vi "niScope Query Trigger Edge.vi"(0 "instrument handle":refnum<k15>, 11 "error in":errorcluster {"code" format="%.0x"}) -> (2 "trigger coupling":i32(slide)=1, 3 "trigger slope":i32(slide), 4 "instrument handle out":refnum<k15>, 6 "trigger source":string(combo)="VAL_IMMEDIATE", 8 "trigger level":dbl format="%.2f", 13 "trigger delay":dbl format="%.4f", 14 "trigger holdoff":dbl format="%.4f", 15 "error out":errorcluster {"code" format="%.0x"})   [LabVIEW 2011]
doc: "This VI configures the common properties of the trigger subsystem. \n\nWhen you call niScope Read Waveform or niScope Initiate Acquisition, the oscilloscope waits for a trigger. You specify the type of trigger for which the oscilloscope waits with the Trigger Type parameter. You specify the source the oscilloscope monitors for the trigger with the Trigger Source parameter. After the oscilloscope receives the trigger, the oscilloscope waits the length of time you specify with the Trigger Delay parameter and then marks this spot as the Reference. The value you specify with the Reference Position parameter of niScope Configure Horizontal determines where the Reference is positioned in a record relative to the start of that record.\n\nIf the oscilloscope is configured to acquire multiple records, it waits the length of time specified with Trigger Holdoff after each record before the trigger system is set to trigger for the next record.\n\nNotes:\n(1) After you call this function, you must call the trigger configuration VI that corresponds to the Trigger Type you select to completely specify the trigger. These configuration functions are niScope Configure Digital Trigger, niScope Configure Edge Trigger, niScope Configure Hysteresis Trigger, niScope Configure TV Trigger, and niScope Configure Window Trigger."
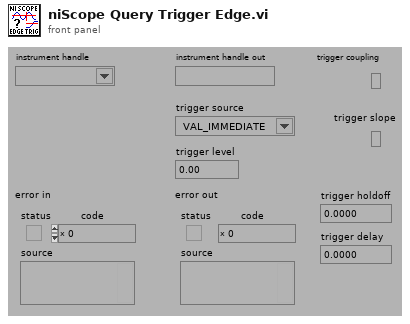
[diagram p1: front panel]
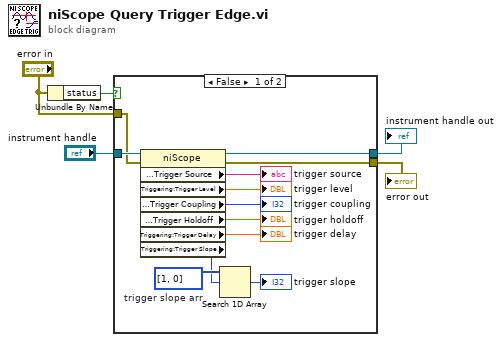
[diagram p0: block diagram]
diagram:
  n1 = Unbundle By Name("error in") -> ("status"=w4:bool)
  n2 = case shown="False" w4 {
    tunnel: "error in" -> [w16 w19]
    tunnel: [w7 w19] -> w3
    tunnel: "instrument handle" -> [w17 w18]
    tunnel: [w6 w18] -> w1
    frame False {
      w15 = i32[] [1, 0]  # trigger slope arr
      n3 = property class="niScope"(reference=w17, error in=w16) -> (reference out=w6:refnum<k15>, error out=w7:errorcluster, "Triggering:Trigger Source"=→"trigger source":string, "Triggering:Trigger Level"=→"trigger level":dbl, "Triggering:Trigger Coupling"=→"trigger coupling":i32, "Triggering:Trigger Holdoff"=→"trigger holdoff":dbl, "Triggering:Trigger Delay"=→"trigger delay":dbl, "Triggering:Trigger Slope"=w14:i32)
      n4 = Search 1D Array(1D array=w15, element=w14) -> (index of element=→"trigger slope":i32)  [unwired: 1 in]
    }
    frame True {
    }
  }
  "error out" <- w3
  "instrument handle out" <- w1
